vi "GE 5565 Write.vi"() -> ()   [LabVIEW 2016]
uses:
  <vilib>/Utility/RT CPU Load.ctl
  <vilib>/Platform/TimedLoop/XDataNode/timing_clust.ctl
  <vilib>/Platform/TimedLoop/XDataNode/nitl_modes.ctl
  <vilib>/Platform/TimedLoop/XDataNode/wakeup.ctl
  <instrlib>/GE 5565 PIORC/Public/DMA Interrupt/GE5565 DMA Read Interrupt (U8) Cluster.vi
  <vilib>/Platform/TimedLoop/XDataNode/XDataNode.xnode
  <instrlib>/GE 5565 PIORC/GE 5565 PIORC.lvlib
  <vilib>/Platform/TimedLoop/XDataNode/XDNodeRunTimeDep.lvlib
  <vilib>/NI_Real-Time Target Support.lvlib
panel:
  out "Times":cluster{u32, u32}
  out "CPU loads":T1[](array[typedef]) {"ISR (%)" format="%#.2f"; "Idle (%)" format="%#.2f"; "Background (%)" format="%#.2f"; "Normal (%)" format="%#.2f"; "Above Normal (%)" format="%#.2f"; "High (%)" format="%#.2g"; "Timed Structures (%)" format="%#.2g"; "Time Critical (%)" format="%#.2g"; "Total (%)" format="%#.2g"}
  in  "mode":enum16{"write", "read"}(ring)
  in  "size":i32=10000
  out "r element":dbl
  in  "r index":i32
  out "r period":u32
  in  "w element":dbl
  in  "w index":i32
  in  "stop":bool
  out "w period":u32
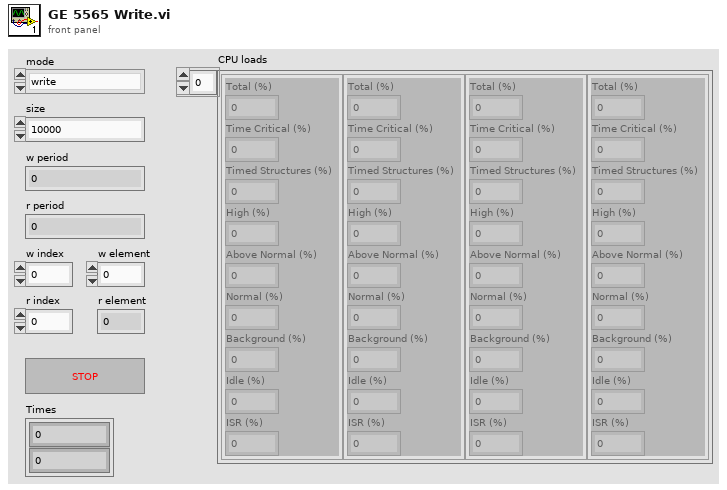
[diagram p1: front panel]
types:
  T1 = typedef "NI_Real-Time Target Support.lvlib/RT CPU Load.ctl" = cluster{"Total (%)":dbl, "Time Critical (%)":dbl, "Timed Structures (%)":dbl, "High (%)":dbl, "Above Normal (%)":dbl, "Normal (%)":dbl, "Background (%)":dbl, "Idle (%)":dbl, "ISR (%)":dbl}
  T2 = typedef "XDNodeRunTimeDep.lvlib/timing_clust.ctl" = cluster{"Expected End [f-1]":u64, "Actual End [f-1]":u64, "Finished Late? [f-1]":bool, "Expected End [i-1]":u64, "Actual End [i-1]":u64, "Finished Late? [i-1]":bool, "Expected Start [i]":u64, "Actual Start [i]":u64, "Expected Start [f]":u64, "Actual Start [f]":u64, "Source Name":string, "Structure Name":string, "Period":i64, "Deadline":i64, "Offset":i64, "Start":i64, "Priority":i32, "Timeout":i32, "Mode":T3, "Wakeup Reason":T4, "Error":errorcluster, "Source Type":string, "Secondary Source Type":string, "Global End Time":u64, "Global Start Time":u64, "Frame Duration":u64, "Iteration Duration":u64, "Assigned CPU":i32, "I/O Scan Engine Mode":u32}
  T3 = typedef "XDNodeRunTimeDep.lvlib/nitl_modes.ctl" = enum32{"No Change", "Process missed periods, maintain original phase", "Discard missed periods, maintain original phase", "Process missed periods, ignore original phase", "Discard missed periods, ignore original phase"}
  T4 = typedef "XDNodeRunTimeDep.lvlib/wakeup.ctl" = enum32{"Normal", "Aborted", "Asynchronous wakeup", "Timing source error", "Timed loop error", "Timeout"}
  T5 = cluster{"VMIC 5565 Resource":refnum<visa-resource-name>, "MEMACC Resource":refnum<visa-resource-name>, "byte count":u32, "mem offset":u32}
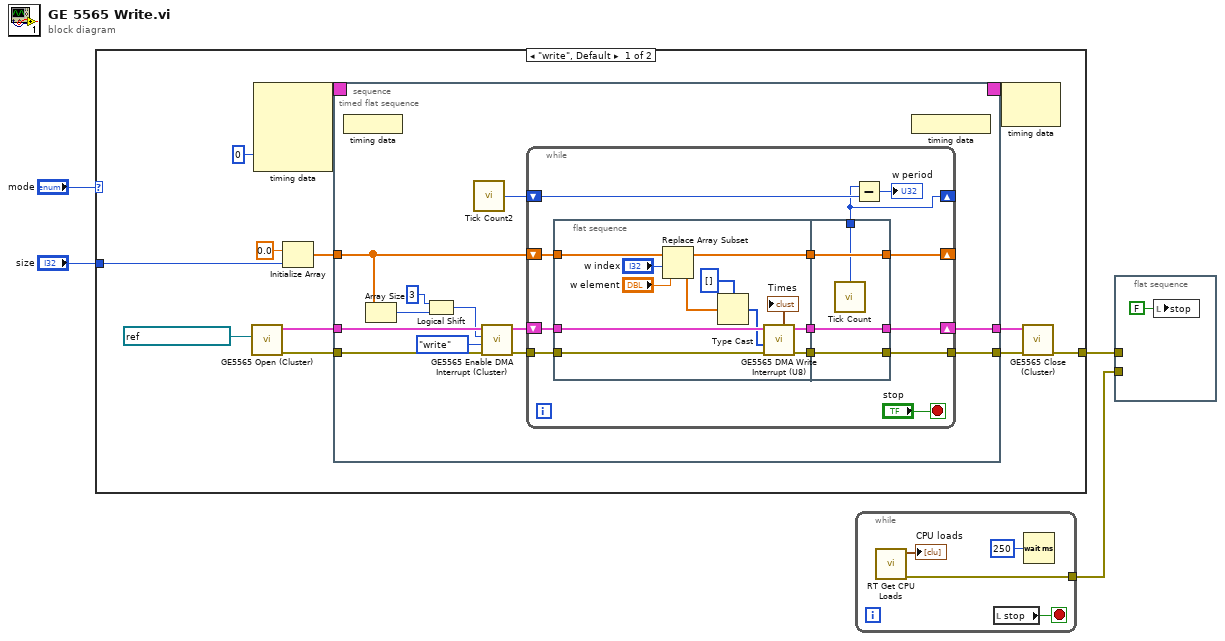
[diagram p0: block diagram]
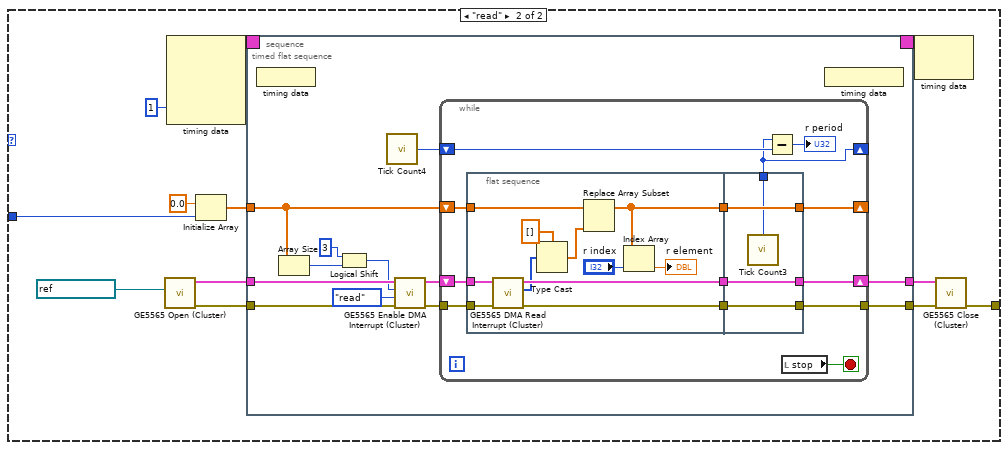
[diagram p2: hidden frame]
diagram:
  n1 = case shown="\"write\", Default" "mode" {
    tunnel: "size" -> [w14 w69]
    tunnel: [w5 w68] -> w2
    frame "write", Default {
      n2 = call <instrlib>:"GE5565 Open (Cluster).vi"("VISA resource name (empty)"=refnum<visa-resource-name> "PXI5::10::INSTR") -> ("error out"=w11:errorcluster, "VMIC-5565"=w12:T5)  [unwired: 5 in]
      n3 = node-c288(0 ("Processor")) -> (w16:T2)  [unwired: 3 in]
      n4 = Initialize Array(0.0 ("element"), w14) -> (w7:dbl[])
      n5 = timed-sequence {
        timing: w16 -> [_]
        timing-out: [_] -> w15
        tunnel: w12 -> [w21]
        tunnel: w11 -> [w20]
        tunnel: [w19] -> w10
        tunnel: [w18] -> w9
        tunnel: w7 -> [w17]
        n6 = timed-flat-sequence {
          tunnel: w21 -> [w33]
          tunnel: w20 -> [w32]
          tunnel: [w30] -> w19
          tunnel: [w28] -> w18
          tunnel: w17 -> [w27]
          n7 = node-c288() -> ()  [unwired: 1 in]
          n8 = Array Size(array=w27) -> (size(s)=w26:i32)
          n9 = Logical Shift(y=i16 3, x=w26) -> (x << y=w24:i32)
          n10 = call "Tick Count2"() -> ("Tick Count(uSec)"=w22:u32)
          n11 = call <instrlib>:"GE5565 Enable DMA Interrupt (Cluster).vi"("error in (no error)"=w32, "operation (read)"=enum16{"read", "write"}."write", "transfer size (1024 bytes)"=w24, "VMIC reference in"=w33) -> ("error out"=w29:errorcluster, "VMIC reference out"=w31:T5)  [unwired: 2 in]
          n12 = while {
            shift-right: [w44] -> w30
            shift-left: w31 -> [w46]
            tunnel: w29 -> [w45]
            tunnel: [w43] -> w28
            shift-right: [w39] -> _
            shift-left: w27 -> [w42]
            shift-right: [w35] -> _
            shift-left: w22 -> [w38]
            stop <- "stop" stop-if-true
            n13 = flat-sequence {
              tunnel: w46 -> [w52]
              tunnel: w45 -> [w51]
              tunnel: w42 -> [w56]
              tunnel: [w50] -> w41
              tunnel: [w55] -> w40
              tunnel: [w49] -> w34
              tunnel: [w59] -> w39
              tunnel: [w60] -> w43
              tunnel: [w61] -> w44
              tunnel: w41 -> [w60]
              tunnel: w40 -> [w59]
              tunnel: [w58] -> w35
              tunnel: w34 -> [w61]
              frame #0 {
                n14 = Replace Array Subset(array=w56, new element="w element", index="w index") -> (w55:dbl[])
                n15 = Type Cast(type=u8[] [], x=w55) -> (*(type *) &x=w48:u8[])
                n16 = call "GE5565 DMA Write Interrupt (U8).vi"("error in (no error)"=w51, "buffer"=w48, "VMIC reference in"=w52) -> ("error out"=w50:errorcluster, "VMIC reference out"=w49:T5, "Times"=→"Times":cluster{u32, u32})  [unwired: 6 in]
              }
              frame #1 {
                n17 = call "Tick Count"() -> ("Tick Count(uSec)"=w58:u32)
              }
            }
            n18 = Subtract(x=w35, y=w38) -> (x-y=→"w period":u32)
          }
          n19 = node-c288() -> ()  [unwired: 1 out]
        }
      }
      n20 = node-c288(w15) -> ()  [unwired: 1 out]
      n21 = call <instrlib>:"GE5565 Close (Cluster).vi"("error in (no error)"=w9, "VMIC reference in"=w10) -> ("error out"=w5:errorcluster)  [unwired: 5 in]
    }
    frame "read" {
      n22 = call <instrlib>:"GE5565 Open (Cluster).vi"("VISA resource name (empty)"=refnum<visa-resource-name> "RefMem2") -> ("error out"=w75:errorcluster, "VMIC-5565"=w76:T5)  [unwired: 5 in]
      n23 = node-c288(1 ("Processor")) -> (w79:T2)  [unwired: 3 in]
      n24 = Initialize Array(0.0 ("element"), w69) -> (w71:dbl[])
      n25 = timed-sequence {
        timing: w79 -> [_]
        timing-out: [_] -> w78
        tunnel: w76 -> [w84]
        tunnel: w75 -> [w83]
        tunnel: [w82] -> w74
        tunnel: [w81] -> w73
        tunnel: w71 -> [w80]
        n26 = timed-flat-sequence {
          tunnel: w84 -> [w96]
          tunnel: w83 -> [w95]
          tunnel: [w93] -> w82
          tunnel: [w91] -> w81
          tunnel: w80 -> [w90]
          n27 = node-c288() -> ()  [unwired: 1 in]
          n28 = Array Size(array=w90) -> (size(s)=w89:i32)
          n29 = Logical Shift(y=i16 3, x=w89) -> (x << y=w87:i32)
          n30 = call "Tick Count4"() -> ("Tick Count(uSec)"=w85:u32)
          n31 = call <instrlib>:"GE5565 Enable DMA Interrupt (Cluster).vi"("error in (no error)"=w95, "operation (read)"=enum16{"read", "write"}."read", "transfer size (1024 bytes)"=w87, "VMIC reference in"=w96) -> ("error out"=w92:errorcluster, "VMIC reference out"=w94:T5)  [unwired: 2 in]
          n32 = while {
            shift-right: [w107] -> w93
            shift-left: w94 -> [w109]
            tunnel: w92 -> [w108]
            tunnel: [w106] -> w91
            shift-right: [w101] -> _
            shift-left: w90 -> [w105]
            shift-right: [w98] -> _
            shift-left: w85 -> [w100]
            stop <- w97 stop-if-true
            n33 = flat-sequence {
              tunnel: w109 -> [w119]
              tunnel: w108 -> [w117]
              tunnel: w105 -> [w114]
              tunnel: [w116] -> w104
              tunnel: [w118] -> w103
              tunnel: [w110] -> w102
              tunnel: [w122] -> w101
              tunnel: [w123] -> w106
              tunnel: [w124] -> w107
              tunnel: w104 -> [w124]
              tunnel: w103 -> [w123]
              tunnel: w102 -> [w122]
              tunnel: [w121] -> w98
              frame #0 {
                n34 = call-poly <instrlib>:"GE5565 DMA Read Interrupt (Cluster).vi"("error in (no error)"=w117, "VMIC reference in"=w119) -> ("error out"=w118:errorcluster, "buffer"=w115:u8[], "VMIC reference out"=w116:T5)  [unwired: 7 in]
                n35 = Type Cast(type=dbl[] [], x=w115) -> (*(type *) &x=w113:dbl[])
                n36 = Replace Array Subset(array=w114, new element=w113) -> (w110:dbl[])  [unwired: 1 in]
                n37 = Index Array(array=w110, index="r index") -> (element=→"r element":dbl)
              }
              frame #1 {
                n38 = call "Tick Count3"() -> ("Tick Count(uSec)"=w121:u32)
              }
            }
            n39 = Subtract(x=w98, y=w100) -> (x-y=→"r period":u32)
            n40 = local read "stop"() -> (w97:bool)
          }
          n41 = node-c288() -> ()  [unwired: 1 out]
        }
      }
      n42 = node-c288(w78) -> ()  [unwired: 1 out]
      n43 = call <instrlib>:"GE5565 Close (Cluster).vi"("error in (no error)"=w73, "VMIC reference in"=w74) -> ("error out"=w68:errorcluster)  [unwired: 5 in]
    }
  }
  n44 = while {
    tunnel: [w131] -> w1
    stop <- w134 stop-if-true
    n45 = call <vilib>:"RT Get CPU Loads.vi"() -> ("error out"=w131:errorcluster, "CPU loads"=→"CPU loads":T1[])  [unwired: 10 in]
    n46 = local read "stop"() -> (w134:bool)
    n47 = Wait (ms)(milliseconds to wait=u32 250) -> ()  [unwired: 1 out]
  }
  n48 = flat-sequence {
    tunnel: w2 -> [_]
    tunnel: w1 -> [_]
    frame #0 {
      n49 = local write "stop"(FALSE ("stop")) -> ()
    }
  }
